vi "Write 8 Bytes.vi"(7 "1-Wire DIO Pin":refnum<k21>="ConnectorA/DIO15", 8 "error in":errorcluster, 10 "Tx data":u64) -> (0 "error out":errorcluster)   [LabVIEW 2014, in "Maxim 1-Wire.lvlib"]
doc: "Writes 8 bytes stored in a U64 to the 1-Wire bus"
uses:
  Maxim 1-Wire.lvlib
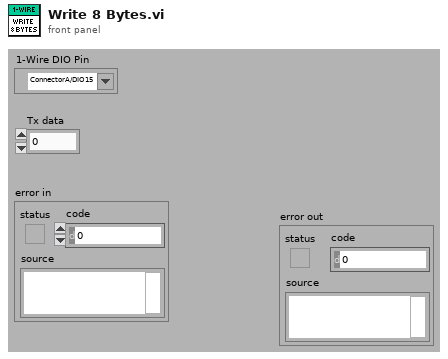
[diagram p1: front panel]
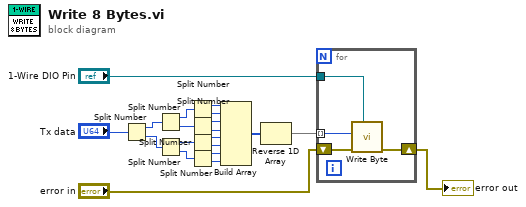
[diagram p0: block diagram]
diagram:
  n1 = Split Number(x="Tx data") -> (hi(x)=w15:u32, lo(x)=w14:u32)
  n2 = Split Number(x=w15) -> (hi(x)=w13:u16, lo(x)=w12:u16)
  n3 = Split Number(x=w14) -> (hi(x)=w11:u16, lo(x)=w10:u16)
  n4 = Split Number(x=w13) -> (hi(x)=w9:u8, lo(x)=w8:u8)
  n5 = Split Number(x=w12) -> (hi(x)=w7:u8, lo(x)=w6:u8)
  n6 = Split Number(x=w11) -> (hi(x)=w5:u8, lo(x)=w4:u8)
  n7 = Split Number(x=w10) -> (hi(x)=w3:u8, lo(x)=w2:u8)
  n8 = Build Array(w9, w8, w7, w6, w5, w4, w3, w2) -> (w1:u8[])
  n9 = Reverse 1D Array(array=w1) -> (reversed array=w16:u8[])
  n10 = for {
    tunnel: "1-Wire DIO Pin" -> [w24]
    tunnel: w16 -> [w21] mode=indexing
    shift-right: [w22] -> w20
    shift-left: "error in" -> [w23]
    n11 = call "Write Byte.vi"("1-Wire DIO Pin"=w24, "error in"=w23, "Tx data"=w21) -> ("error out"=w22:errorcluster)  [unwired: 8 in]
  }
  "error out" <- w20
